vi "Convert Double to String.vi"(1 "Value":dbl) -> (0 "String":string)   [LabVIEW 2018, in "ASI TG-1000.lvlib"]
uses:
  ASI TG-1000.lvlib
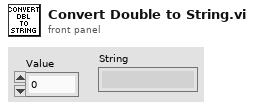
[diagram p1: front panel]
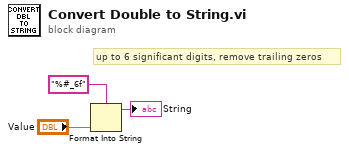
[diagram p0: block diagram]
diagram:
  # "up to 6 significant digits, remove trailing zeros"
  n1 = Format Into String(format string="%#_6f", "Value") -> (resulting string=→"String":string)  [unwired: 2 in, 1 out]
